vi "Export Configuration.vi"(8 "error in (no error)":errorcluster, 11 "Node Ptr":u64 format="%.0x") -> (0 "error out":errorcluster)   [LabVIEW 2014, in "SLSC configuration System Explorer.lvlib"]
uses:
  SLSC configuration System Explorer.lvlib
  U:/NI/Custom VeriStand Development/DET-SPI-Tool/XML Deserializer/SLSC Deserializer/SLSC Deserializer/bin/Release/SLSC Deserializer.dll
  XML Deserializer/SLSC Deserializer/SLSC Deserializer/bin/Release/SLSC Deserializer.dll
panel:
  in  "Cancel":bool
  in  "OK":bool
  in  "XML Export Path":path
  in  "Tag":string
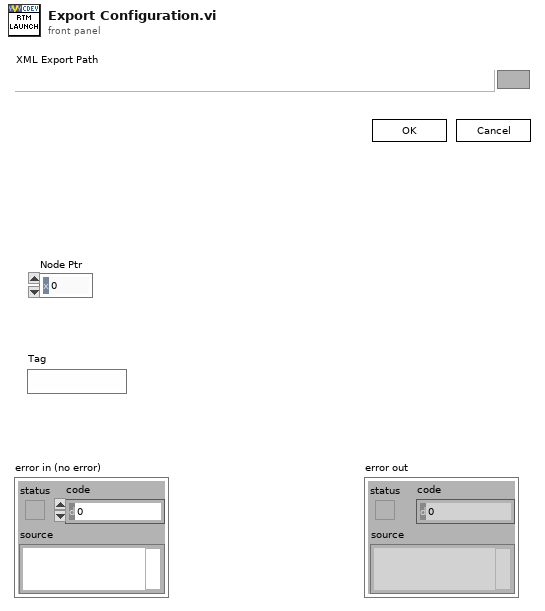
[diagram p1: front panel]
types:
  T1 = enum8{"Enabled", "Disabled", "Disabled and Grayed Out"}
  T2 = typedef "Custom Device API.lvlib/Custom Device Item Ref.ctl" = u64
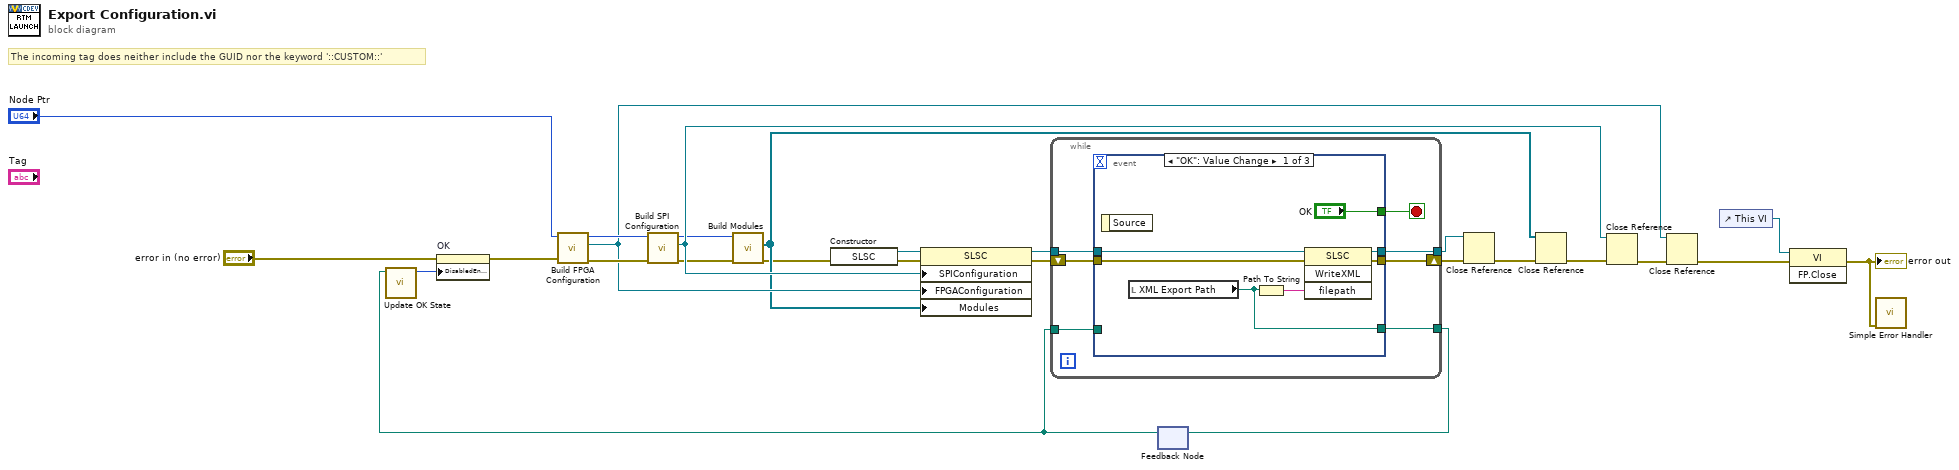
[diagram p0: block diagram]
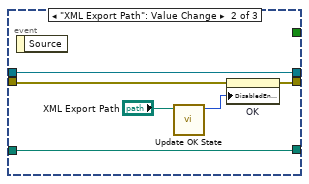
[diagram p2: hidden frame]
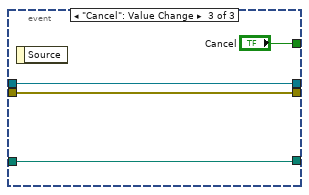
[diagram p3: hidden frame]
diagram:
  # "The incoming tag does neither include the GUID nor the keyword '::CUSTOM::'"
  n1 = feedback #1() -> (w2:path)  [unwired: 1 in]
  n2 = call "Update OK State.vi"("XML Export Path"=w2) -> ("OK State"=w14:T1)  [unwired: 10 in]
  n3 = property on="OK" class="Bool"(error in="error in (no error)", "DisabledEnum"=w14) -> (error out=w12:errorcluster)  [unwired: 1 in, 1 out]
  n4 = call "Build FPGA Configuration.vi"("error in (no error)"=w12, "Item Ref in"="Node Ptr") -> ("error out"=w25:errorcluster, "SLSCFPGAConfiguration"=w15:refnum<k24>, "Item Ref out"=w24:T2)  [unwired: 7 in]
  n5 = call "Build SPI Configuration.vi"("error in (no error)"=w25, "Item Ref in"=w24) -> ("error out"=w9:errorcluster, "SLSCSPIConfiguration"=w17:refnum<k24>, "Item Ref out"=w8:T2)  [unwired: 7 in]
  n6 = call "Build Modules.vi"("error in (no error)"=w9, "Item Ref in"=w8) -> ("error out"=w4:errorcluster, "Modules"=w5:refnum<k24>[])  [unwired: 7 in, 1 out]
  n7 = constructor class="SLSC"(error in=w4) -> (reference out=w22:refnum<k24>, error out=w23:errorcluster)  [unwired: 2 in, 1 out]
  n8 = property class="SLSC"(reference=w22, error in=w23, "SPIConfiguration"=w17, "FPGAConfiguration"=w15, "Modules"=w5) -> (reference out=w20:refnum<k24>, error out=w21:errorcluster)
  n9 = while {
    shift-right: [w30] -> w19
    shift-left: w21 -> [w33]
    tunnel: w20 -> [w31]
    tunnel: [w29] -> w18
    tunnel: [w28] -> w3
    tunnel: w2 -> [w27]
    stop <- w32 stop-if-true
    n10 = event shown="[0] \"OK\": Value Change" {
      selector: _ -> [_ _ _]
      dyn-events: _ -> [_ _ _]
      timeout: _ -> [_ _ _]
      tunnel: w33 -> [w39 w44 w50]
      tunnel: ["OK" _ "Cancel"] -> w32
      tunnel: w31 -> [w38 w45 w49]
      tunnel: [w36 w46 w50] -> w30
      tunnel: [w35 w45 w49] -> w29
      tunnel: [w34 w43 w47] -> w28
      tunnel: w27 -> [_ w43 w47]
      event "OK": Value Change {
        n11 = event-data() -> ()  [unwired: 1 in, 1 out]
        n12 = local read "XML Export Path"() -> (w34:path)
        n13 = Path To String(path=w34) -> (string=w37:string)
        n14 = invoke class="SLSC" method="WriteXML"(reference=w38, error in=w39, "filepath"=w37) -> (reference out=w35:refnum<k24>, error out=w36:errorcluster)  [unwired: 1 in, 2 out]
      }
      event "XML Export Path": Value Change {
        n15 = event-data() -> ()  [unwired: 1 in, 1 out]
        n16 = call "Update OK State.vi"("XML Export Path"="XML Export Path") -> ("OK State"=w41:T1)  [unwired: 10 in]
        n17 = property on="OK" class="Bool"(error in=w44, "DisabledEnum"=w41) -> (error out=w46:errorcluster)  [unwired: 1 in, 1 out]
      }
      event "Cancel": Value Change {
        n18 = event-data() -> ()  [unwired: 1 in, 1 out]
      }
    }
  }
  n19 = feedback-in #1(w3) -> ()
  n20 = Close Reference(reference=w18, error in (no error)=w19) -> (error out=w7:errorcluster)
  n21 = Close Reference(reference=w5, error in (no error)=w7) -> (error out=w6:errorcluster)
  n22 = Close Reference(reference=w17, error in (no error)=w6) -> (error out=w16:errorcluster)
  n23 = Close Reference(reference=w15, error in (no error)=w16) -> (error out=w10:errorcluster)
  n24 = control-ref of="This VI"() -> (w11:refnum<vi>)
  n25 = invoke class="VI" method="FP.Close"(reference=w11, error in=w10) -> (error out=w1:errorcluster)  [unwired: 1 in, 2 out]
  "error out" <- w1
  n26 = call <vilib>:"Simple Error Handler.vi"("error in (no error)"=w1) -> ()  [unwired: 4 in, 5 out]
